vi "PH_AxisGUI_BaseClass.Service2Axis.vi"(0 "i ref in":refnum<vi>, 2 "Service Name":string="N/A", 3 "Tag":T4, 5 "error in":errorcluster) -> (14 "i ref out":refnum<vi>, 16 "Axis":i32=-1, 17 "Axis Data":T1={"Axis GUI Refs"={"Back"=refnum, "Forth"=refnum, "Status"=refnum, "Target"=refnum, "Address"=refnum, "Status Bar"=refnum, "Settings"=refnum, "Activity"=refnum, "Clear Error"=refnum}, "Address"={"Instance"="N/A", "Motor Nr"=0}, "Name"="", "Label \"Back\""="", "Labell \"Forth\""="", "Moving?"=FALSE}, 19 "error out":errorcluster)   [LabVIEW 2014, in "PH_AxisGUI_BaseClass.lvlib"]
doc: "This VI gets the axis number from the service name."
uses:
  PH_AxisGUI_BaseClass.lvlib
  PH_Stepmotor_BaseClass/PH_Stepmotor_BaseClass.Axis DIM Tags.ctl
  PH_AxisGUI_BaseClass.Axis Attributes.ctl
  PH_AxisGUI_BaseClass.Axis GUI Refs.ctl
  PH_Stepmotor_BaseClass/PH_Stepmotor_BaseClass.Axis Address.ctl
  PH_Stepmotor_BaseClass/PH_Stepmotor_BaseClass.Axis Settings.ctl
  PH_Stepmotor_BaseClass/PH_Stepmotor_BaseClass.Motor Type.ctl
  PH_Stepmotor_BaseClass/PH_Stepmotor_BaseClass.Axis Activity.ctl
  PH_Stepmotor_BaseClass/PH_Stepmotor_BaseClass.lvlib
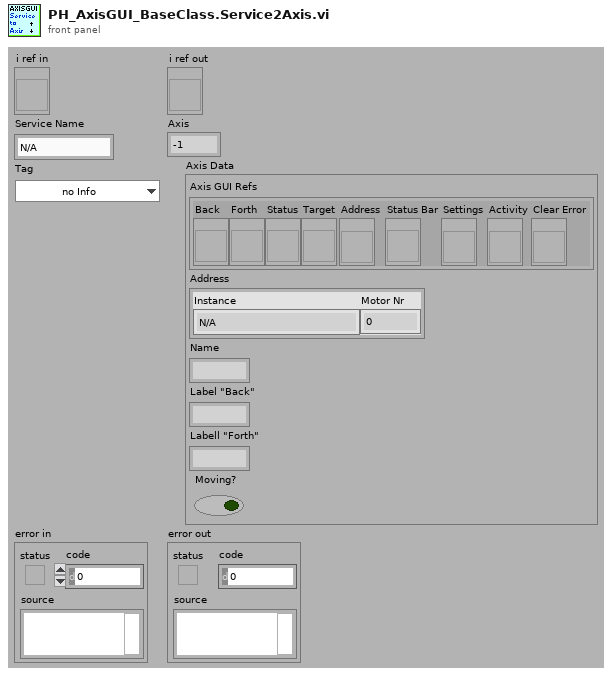
[diagram p1: front panel]
types:
  T1 = typedef "PH_AxisGUI_BaseClass.lvlib/PH_AxisGUI_BaseClass.Axis Attributes.ctl" = cluster{"Axis GUI Refs":T2, "Address":T3, "Name":string, "Label \"Back\"":string, "Labell \"Forth\"":string, "Moving?":bool}
  T2 = typedef "PH_AxisGUI_BaseClass.lvlib/PH_AxisGUI_BaseClass.Axis GUI Refs.ctl" = cluster{"Back":refnum<vi>, "Forth":refnum<vi>, "Status":refnum<vi>, "Target":refnum<vi>, "Address":refnum<vi>, "Status Bar":refnum<vi>, "Settings":refnum<vi>, "Activity":refnum<vi>, "Clear Error":refnum<vi>}
  T3 = typedef "PH_Stepmotor_BaseClass.lvlib/PH_Stepmotor_BaseClass.Axis Address.ctl" = cluster{"Instance":string, "Motor Nr":i32}
  T4 = typedef "PH_Stepmotor_BaseClass.lvlib/PH_Stepmotor_BaseClass.Axis DIM Tags.ctl" = enum16{"no Info", "Information", "Settings"}
  T5 = typedef "PH_AxisGUI_BaseClass.lvlib/PH_AxisGUI_BaseClass.i attribute.ctl" = cluster{"Axes":T1[]}
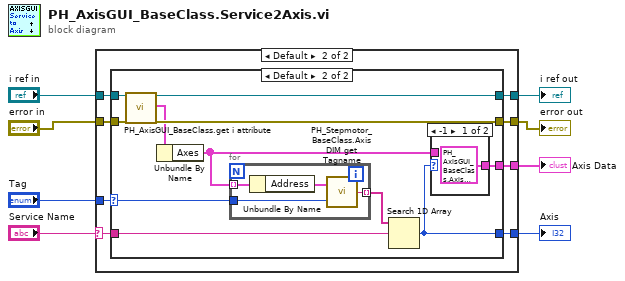
[diagram p0: block diagram]
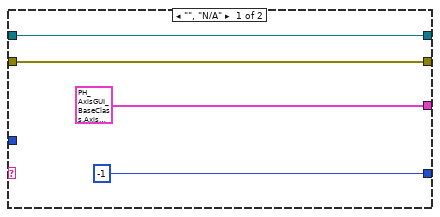
[diagram p2: hidden frame]
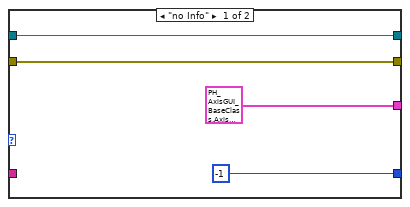
[diagram p3: hidden frame]
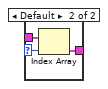
[diagram p4: hidden frame]
diagram:
  n1 = case shown="Default" "Service Name" {
    selector: "Service Name" -> [_ w13]
    tunnel: [w11 w20] -> w8
    tunnel: [w12 w19] -> w7
    tunnel: "error in" -> [w11 w18]
    tunnel: "i ref in" -> [w12 w17]
    tunnel: [T1 {"Axis GUI Refs"={"Back"=refnum, "Forth"=refnum, "Status"=refnum, "Target"=refnum, "Address"=refnum, "Status Bar"=refnum, "Settings"=refnum, "Activity"=refnum, "Clear Error"=refnum}, "Address"={"Instance"="N/A", "Motor Nr"=0}, "Name"="", "Label \"Back\""="", "Labell \"Forth\""="", "Moving?"=FALSE} ("Axis") w16] -> w4
    tunnel: [-1 ("index of element") w15] -> w3
    tunnel: "Tag" -> [_ w14]
    frame "", "N/A" {
    }
    frame Default {
      n2 = case shown="Default" w14 {
        selector: w14 -> [_ w25]
        tunnel: [w22 w35] -> w20
        tunnel: [w21 w34] -> w19
        tunnel: w18 -> [w22 w33]
        tunnel: w17 -> [w21 w32]
        tunnel: w13 -> [_ w31]
        tunnel: [T1 {"Axis GUI Refs"={"Back"=refnum, "Forth"=refnum, "Status"=refnum, "Target"=refnum, "Address"=refnum, "Status Bar"=refnum, "Settings"=refnum, "Activity"=refnum, "Clear Error"=refnum}, "Address"={"Instance"="N/A", "Motor Nr"=0}, "Name"="", "Label \"Back\""="", "Labell \"Forth\""="", "Moving?"=FALSE} ("Axis") w27] -> w16
        tunnel: [-1 ("index of element") w26] -> w15
        frame "no Info" {
        }
        frame Default {
          n3 = call "PH_AxisGUI_BaseClass.get i attribute.vi"("i ref in"=w32, "error in (no error)"=w33) -> ("i ref out"=w34:refnum<vi>, "i attribute"=w29:T5, "error out"=w35:errorcluster)  [unwired: 15 in]
          n4 = Unbundle By Name(w29) -> ("Axes"=w28:T1[])
          n5 = for {
            tunnel: w28 -> [w43] mode=indexing
            tunnel: w25 -> [w42]
            tunnel: [w41] -> w30 mode=indexing
            n6 = Unbundle By Name(w43) -> ("Address"=w40:T3)
            n7 = call "PH_Stepmotor_BaseClass.Axis DIM get Tagname.vi"("Tag"=w42, "Instancename"=w40) -> ("Axis Tagname"=w41:string)
          }
          n8 = Search 1D Array(1D array=w30, element=w31) -> (index of element=w26:i32)  [unwired: 1 in]
          n9 = case shown="-1" w26 {
            selector: w26 -> [_ w37]
            tunnel: w28 -> [_ w39]
            tunnel: [T1 {"Axis GUI Refs"={"Back"=refnum, "Forth"=refnum, "Status"=refnum, "Target"=refnum, "Address"=refnum, "Status Bar"=refnum, "Settings"=refnum, "Activity"=refnum, "Clear Error"=refnum}, "Address"={"Instance"="N/A", "Motor Nr"=0}, "Name"="", "Label \"Back\""="", "Labell \"Forth\""="", "Moving?"=FALSE} ("Axis") w38] -> w27
            frame -1 {
            }
            frame Default {
              n10 = Index Array(array=w39, index=w37) -> (element=w38:T1)
            }
          }
        }
      }
    }
  }
  "error out" <- w8
  "i ref out" <- w7
  "Axis" <- w3
  "Axis Data" <- w4
